vi "A33Trg_py.vi"() -> ()   [LabVIEW 2022 SP3]
uses:
  <vilib>/addons/zeromq/zmq_socket.lvclass
panel:
  out "Standalone":bool
  out "socket out":refnum<class "zmq_socket.lvclass">
  in  "socket in":refnum<class "zmq_socket.lvclass">
  out "error out":errorcluster
  out "resulting string":string
  in  "Instrument":string="AG33600A_Gen1"
  in  "error in (no error)":errorcluster
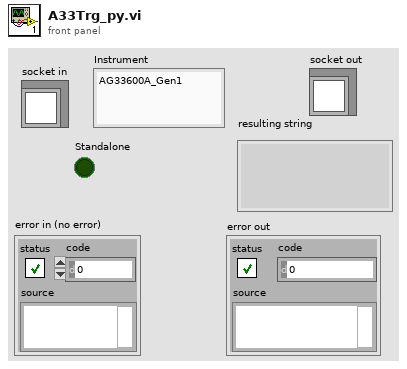
[diagram p1: front panel]
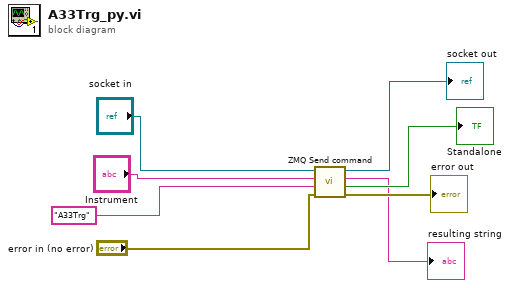
[diagram p0: block diagram]
diagram:
  n1 = call "ZMQ Send command.vi"("error in"="error in (no error)", "Command"="A33Trg", "Instrument"="Instrument", "socket in"="socket in") -> ("error out"=→"error out":errorcluster, "Standalone"=→"Standalone":bool, "Recieved message"=→"resulting string":string, "socket out"=→"socket out":refnum<class "zmq_socket.lvclass">)  [unwired: 4 in]
